vi "Protocol.Create XNET Sessions.vi"(8 "error in (no error)":errorcluster, 11 "Parameters in":T1={"XNET Settings"={"Database"="", "Cluster"="", "Port"="", "Baud rate [Bd]"=0, "Termination"=0, "Incoming Rate"=0, "Outcoming Rate"=1, "Write Decimation"=1}, "Data"=[], "DTCs"=[], "Sim Addresses LUT"=variant, "Data Table LUT"=variant, "MonitorTool.Network"={"Address"=0, "Name"=0}, "Name"=""} {"MonitorTool.Network"."Name" format="%.0x"; "DTCs"."Data"."DM1 Ref"."Data Reference" format="%.0x"; "DTCs"."Data"."DM1 Enable Ref"."Data Reference" format="%.0x"; "DTCs"."Data"."DM2 Ref"."Data Reference" format="%.0x"; "DTCs"."Data"."DM2 Enable Ref"."Data Reference" format="%.0x"; "Data"."Trigger.Refs"."Data Reference" format="%.0x"; "Data"."Disable.Refs"."Data Reference" format="%.0x"; "Data"."Timing.Refs"."Data Reference" format="%.0x"; "Data"."Network"."Name" format="%.0x"; "Data"."Incoming.Refs"."Data Reference" format="%.0x"; "Data"."Outgoing.Refs"."Data Reference" format="%.0x"; "XNET Settings"."Termination" items=["Off", "On"]}) -> (0 "error out":errorcluster, 3 "XNET":T12)   [LabVIEW 2015, in "J1939 Addon Engine.lvlib"]
uses:
  J1939 Addon Engine.lvlib
  Types/Protocol.XNET Settings.ctl
  Types/Protocol.App Settings.ctl
  Shared/Types/XNET Settings.ctl
  Types/Protocol.XNET Refs.ctl
  Shared/Types/Monitor Settings.ctl
  <vilib>/NI Veristand/Custom Device API/Block Data Reference.ctl
  <vilib>/NI Veristand/Custom Device API/Data Reference.ctl
  Types/Main.Outgoing.Frame.Settings.ctl
  Shared/Types/Outgoing Event Trigger Types.ctl
  Types/Engine.DTC Settings.ctl
  Shared/Types/Compiled Simulated Settings.ctl
  Types/Engine.DTC FIFOs.ctl
  <vilib>/xnet/xnet.llb/XNET Control Scope.ctl
  <vilib>/xnet/xnet.llb/XNET Create Session (Frame Output Stream).vi
  <vilib>/xnet/xnet.llb/XNET Create Session (Frame Input Stream).vi
  <resource>/objmgr/xnet.rc
  Shared/J1939 Addon Shared.lvlib
  <vilib>/NI VeriStand/Custom Device API/Custom Device API.lvlib
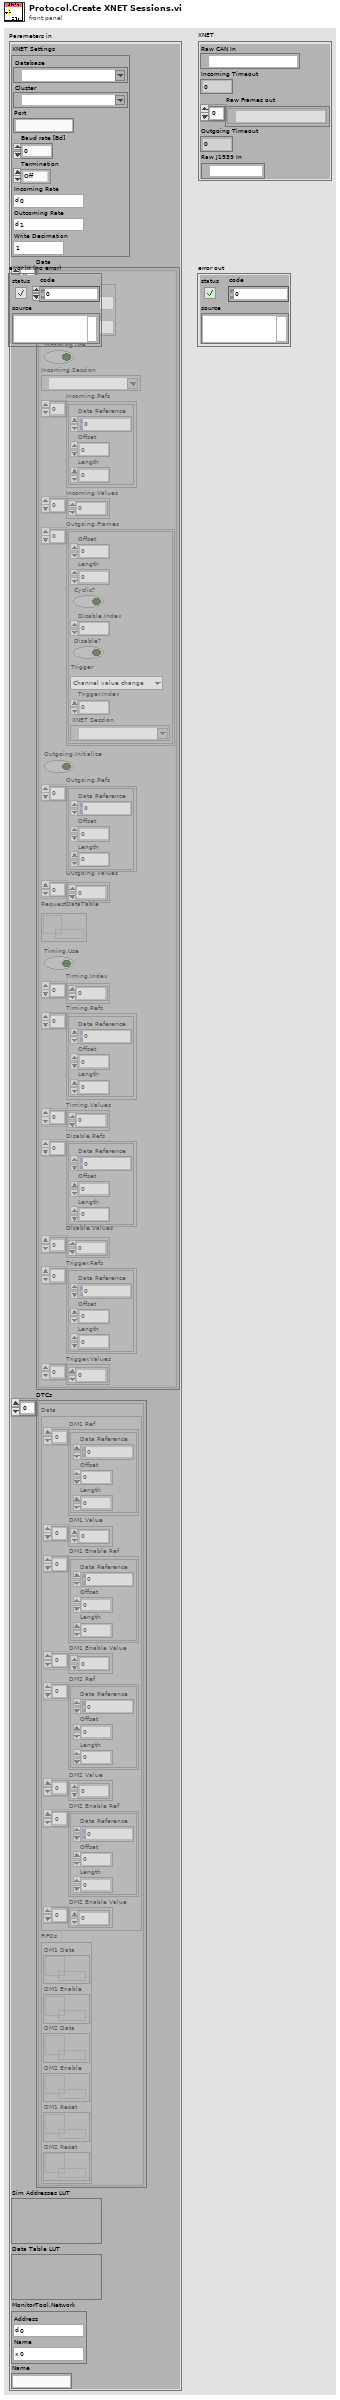
[diagram p1: front panel]
types:
  T1 = typedef "J1939 Addon Engine.lvlib/Protocol.App Settings.ctl" = cluster{"XNET Settings":T2, "Data":T3[], "DTCs":T9[], "Sim Addresses LUT":variant, "Data Table LUT":variant, "MonitorTool.Network":T4, "Name":string}
  T2 = typedef "J1939 Addon Shared.lvlib/XNET Settings.ctl" = cluster{"Database":refnum<k21>, "Cluster":refnum<k21>, "Port":string, "Baud rate [Bd]":u32, "Termination":u32, "Incoming Rate":u32, "Outcoming Rate":u32, "Write Decimation":u32}
  T3 = typedef "J1939 Addon Engine.lvlib/Protocol.XNET Refs.ctl" = cluster{"Network":T4, "Incoming.Use":bool, "Incoming.Session":refnum<k21>, "Incoming.Refs":T5[], "Incoming.Values":dbl[], "Outgoing.Frames":T7[], "Outgoing.Initialize":bool, "Outgoing.Refs":T5[], "Outgoing.Values":dbl[], "RequestDataTable":refnum<k33>, "Timing.Use":bool, "Timing.Index":i32[], "Timing.Refs":T5[], "Timing.Values":dbl[], "Disable.Refs":T5[], "Disable.Values":dbl[], "Trigger.Refs":T5[], "Trigger.Values":dbl[]}
  T4 = typedef "J1939 Addon Shared.lvlib/Monitor Settings.ctl" = cluster{"Address":u8, "Name":u64}
  T5 = typedef "Custom Device API.lvlib/Block Data Reference.ctl" = cluster{"Data Reference":T6, "Offset":u64, "Length":u64}
  T6 = typedef "Custom Device API.lvlib/Data Reference.ctl" = i32
  T7 = typedef "J1939 Addon Engine.lvlib/Main.Outgoing.Frame.Settings.ctl" = cluster{"Offset":u32, "Length":u32, "Cyclic?":bool, "Disable.Index":i32, "Disable?":bool, "Trigger":T8, "Trigger.Index":i32, "XNET Session":refnum<k21>}
  T8 = typedef "J1939 Addon Shared.lvlib/Outgoing Event Trigger Types.ctl" = enum16{"Channel value change", "Trigger channel (not zero)", "Channel value change or trigger channel (not zero)", "Trigger channel (any value change)", "Channel value change or trigger channel (any value change)"}
  T9 = typedef "J1939 Addon Engine.lvlib/Engine.DTC Settings.ctl" = cluster{"Data":T10, "FIFOs":T11}
  T10 = typedef "J1939 Addon Shared.lvlib/Compiled Simulated Settings.ctl" = cluster{"DM1 Ref":T5[], "DM1 Value":dbl[], "DM1 Enable Ref":T5[], "DM1 Enable Value":dbl[], "DM2 Ref":T5[], "DM2 Value":dbl[], "DM2 Enable Ref":T5[], "DM2 Enable Value":dbl[]}
  T11 = typedef "J1939 Addon Engine.lvlib/Engine.DTC FIFOs.ctl" = cluster{"DM1 Data":refnum<k33>, "DM1 Enable":refnum<k33>, "DM2 Data":refnum<k33>, "DM2 Enable":refnum<k33>, "DM1 Reset":refnum<k33>, "DM2 Reset":refnum<k33>}
  T12 = typedef "J1939 Addon Engine.lvlib/Protocol.XNET Settings.ctl" = cluster{"Raw CAN In":refnum<k21>, "Incoming Timeout":u32, "Raw Frames out":refnum<k21>[], "Outgoing Timeout":u32, "Raw J1939 In":refnum<k21>}
  T13 = typedef "XNET Control Scope.ctl" = u32
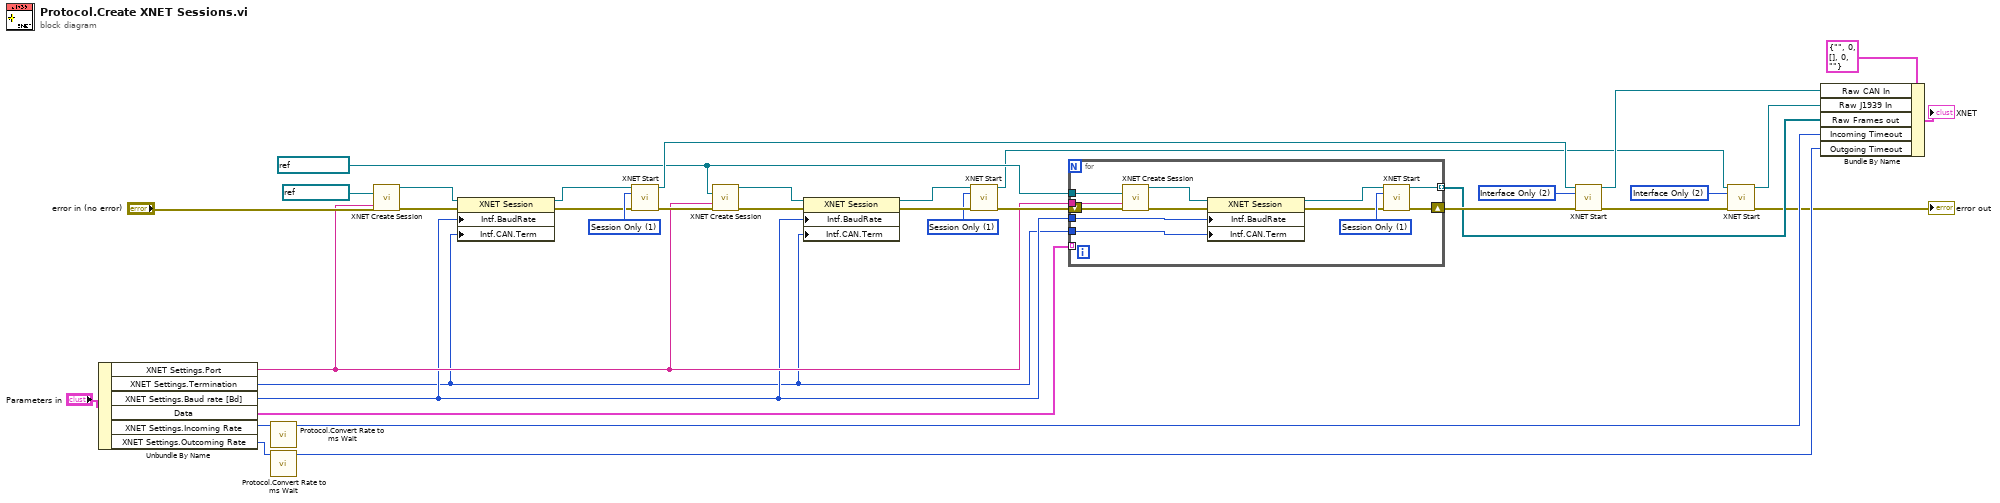
[diagram p0: block diagram]
diagram:
  w5 = T13 2 items=["Normal", "Session Only", "Interface Only", "Session Only Blocking"] ("scope (normal)")
  w15 = T13 1 items=["Normal", "Session Only", "Interface Only", "Session Only Blocking"] ("scope (normal)")
  w23 = T13 2 items=["Normal", "Session Only", "Interface Only", "Session Only Blocking"] ("scope (normal)")
  w26 = T13 1 items=["Normal", "Session Only", "Interface Only", "Session Only Blocking"] ("scope (normal)")
  w9 = refnum<k21> ":can_j1939:" ("cluster (:memory:)")
  n1 = Unbundle By Name("Parameters in") -> ("XNET Settings.Port"=w8:string, "XNET Settings.Termination"=w6:u32, "XNET Settings.Baud rate [Bd]"=w7:u32, "Data"=w19:T3[], "XNET Settings.Incoming Rate"=w31:u32, "XNET Settings.Outcoming Rate"=w32:u32)
  n2 = call "Protocol.Convert Rate to ms Wait.vi"("Rate"=w31) -> ("ms"=w35:u32)  [unwired: 10 in]
  n3 = call "Protocol.Convert Rate to ms Wait.vi"("Rate"=w32) -> ("ms"=w34:u32)  [unwired: 10 in]
  n4 = call-poly <vilib>:"XNET Create Session.vi"("cluster (:memory:)"=refnum<k21> ":memory:", "interface"=w8, "error in (no error)"="error in (no error)") -> ("session out"=w28:refnum<k21>, "error out"=w29:errorcluster)  [unwired: 11 out]
  n5 = property class="XNET Session"(reference=w28, error in=w29, "Intf.BaudRate"=w7, "Intf.CAN.Term"=w6) -> (reference out=w24:refnum<k21>, error out=w25:errorcluster)
  n6 = call <vilib>:"XNET Start.vi"("session in"=w24, "scope (normal)"=w26, "error in (no error)"=w25) -> ("session out"=w21:refnum<k21>, "error out"=w13:errorcluster)  [unwired: 11 in]
  n7 = call-poly <vilib>:"XNET Create Session.vi"("cluster (:memory:)"=w9, "interface"=w8, "error in (no error)"=w13) -> ("session out"=w10:refnum<k21>, "error out"=w14:errorcluster)  [unwired: 11 out]
  n8 = property class="XNET Session"(reference=w10, error in=w14, "Intf.BaudRate"=w7, "Intf.CAN.Term"=w6) -> (reference out=w11:refnum<k21>, error out=w16:errorcluster)
  n9 = call <vilib>:"XNET Start.vi"("session in"=w11, "scope (normal)"=w15, "error in (no error)"=w16) -> ("session out"=w2:refnum<k21>, "error out"=w12:errorcluster)  [unwired: 11 in]
  n10 = for {
    tunnel: [w37] -> w18 mode=indexing
    tunnel: w7 -> [w48]
    tunnel: w6 -> [w47]
    tunnel: w8 -> [w46]
    tunnel: w9 -> [w43]
    shift-right: [w39] -> w22
    shift-left: w12 -> [w42]
    tunnel: w19 -> [_] mode=indexing
    w41 = T13 1 items=["Normal", "Session Only", "Interface Only", "Session Only Blocking"] ("scope (normal)")
    n11 = call-poly <vilib>:"XNET Create Session.vi"("cluster (:memory:)"=w43, "interface"=w46, "error in (no error)"=w42) -> ("session out"=w44:refnum<k21>, "error out"=w45:errorcluster)  [unwired: 11 out]
    n12 = property class="XNET Session"(reference=w44, error in=w45, "Intf.BaudRate"=w48, "Intf.CAN.Term"=w47) -> (reference out=w38:refnum<k21>, error out=w40:errorcluster)
    n13 = call <vilib>:"XNET Start.vi"("session in"=w38, "scope (normal)"=w41, "error in (no error)"=w40) -> ("session out"=w37:refnum<k21>, "error out"=w39:errorcluster)  [unwired: 11 in]
  }
  n14 = call <vilib>:"XNET Start.vi"("session in"=w21, "scope (normal)"=w23, "error in (no error)"=w22) -> ("session out"=w20:refnum<k21>, "error out"=w4:errorcluster)  [unwired: 11 in]
  n15 = call <vilib>:"XNET Start.vi"("session in"=w2, "scope (normal)"=w5, "error in (no error)"=w4) -> ("session out"=w1:refnum<k21>, "error out"=→"error out":errorcluster)  [unwired: 11 in]
  n16 = Bundle By Name(cluster=T12 {"Raw CAN In"="", "Incoming Timeout"=0, "Raw Frames out"=[], "Outgoing Timeout"=0, "Raw J1939 In"=""} ("XNET"), "Raw CAN In"=w20, "Raw J1939 In"=w1, "Raw Frames out"=w18, "Incoming Timeout"=w35, "Outgoing Timeout"=w34) -> (→"XNET":T12)
